vi "prop_axes_prop_to_page.vi"(10 "Axes Properties":T2) -> (2 "Axes Property Page":T1(array[cluster]))   [LabVIEW 2020, in "3DPC_SurfacePlot.xctl"]
uses:
  <vilib>/Native 3D Graph/xcontrol/3DPC_SurfacePlot.xctl
  <vilib>/Native 3D Graph/typedefs/prop_axes_all.ctl
  <vilib>/Native 3D Graph/typedefs/prop_axes_grid.ctl
  <vilib>/Native 3D Graph/typedefs/prop_axes_ticks.ctl
  <vilib>/Native 3D Graph/typedefs/range_cluster.ctl
  <vilib>/Native 3D Graph/typedefs/min_max.ctl
  <vilib>/Native 3D Graph/typedefs/prop_axes_captions.ctl
  <vilib>/Native 3D Graph/typedefs/prop_axes_labels.ctl
  <vilib>/Native 3D Graph/typedefs/prop_axes_autorange.ctl
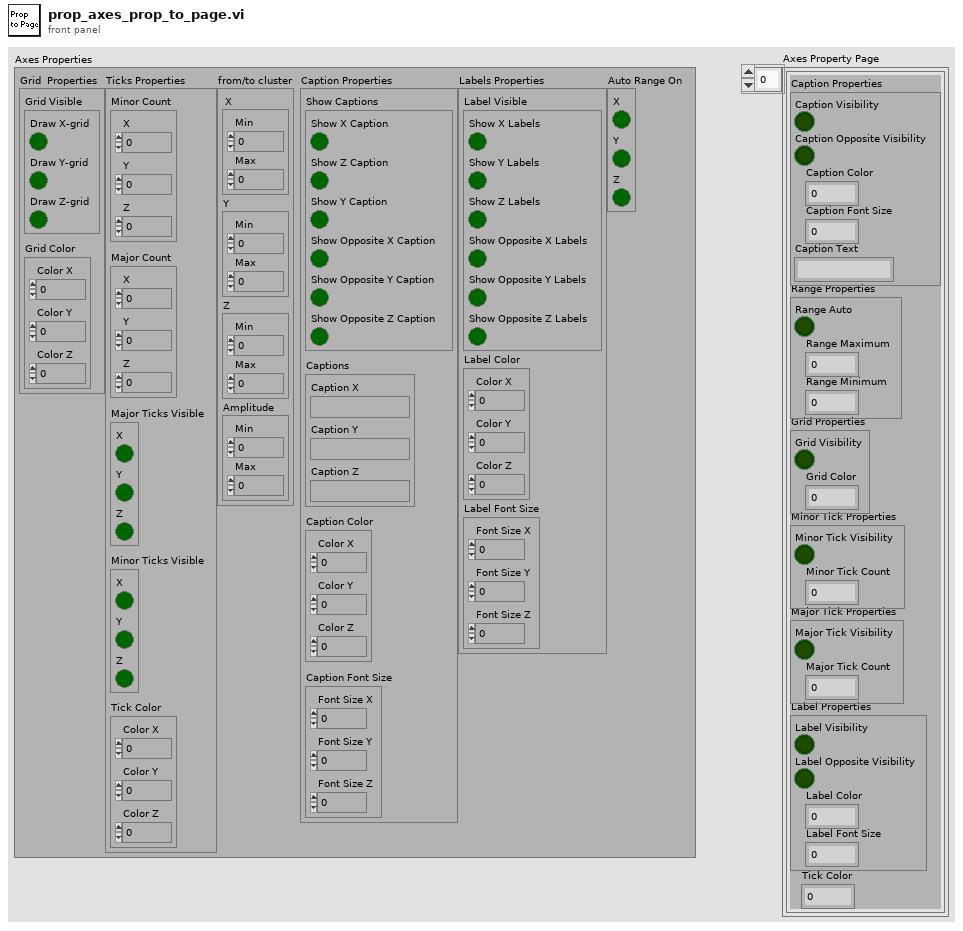
[diagram p1: front panel]
types:
  T1 = cluster{"Caption Properties":cluster{"Caption Visibility":bool, "Caption Opposite Visibility":bool, "Caption Color":u32, "Caption Font Size":i32, "Caption Text":string}, "Range Properties":cluster{"Range Auto":bool, "Range Maximum":dbl, "Range Minimum":dbl}, "Grid Properties":cluster{"Grid Visibility":bool, "Grid Color":u32}, "Minor Tick Properties":cluster{"Minor Tick Visibility":bool, "Minor Tick Count":i32}, "Major Tick Properties":cluster{"Major Tick Visibility":bool, "Major Tick Count":i32}, "Label Properties":cluster{"Label Visibility":bool, "Label Opposite Visibility":bool, "Label Color":u32, "Label Font Size":i32}, "Tick Color":u32}[]
  T2 = typedef "3DPC_SurfacePlot.xctl/prop_axes_all.ctl" = cluster{"Grid  Properties":T3, "Ticks Properties":T4, "from/to cluster":T5, "Caption Properties":T7, "Labels Properties":T8, "Auto Range On":T9}
  T3 = typedef "3DPC_SurfacePlot.xctl/prop_axes_grid.ctl" = cluster{"Grid Visible":cluster{"Draw X-grid":bool, "Draw Y-grid":bool, "Draw Z-grid":bool}, "Grid Color":cluster{"Color X":u32, "Color Y":u32, "Color Z":u32}}
  T4 = typedef "3DPC_SurfacePlot.xctl/prop_axes_ticks.ctl" = cluster{"Minor Count":cluster{"X":i32, "Y":i32, "Z":i32}, "Major Count":cluster{"X":i32, "Y":i32, "Z":i32}, "Major Ticks Visible":cluster{"X":bool, "Y":bool, "Z":bool}, "Minor Ticks Visible":cluster{"X":bool, "Y":bool, "Z":bool}, "Tick Color":cluster{"Color X":u32, "Color Y":u32, "Color Z":u32}}
  T5 = typedef "3DPC_SurfacePlot.xctl/range_cluster.ctl" = cluster{"X":T6, "Y":T6, "Z":T6, "Amplitude":T6}
  T6 = typedef "3DPC_SurfacePlot.xctl/min_max.ctl" = cluster{"Min":sgl, "Max":sgl}
  T7 = typedef "3DPC_SurfacePlot.xctl/prop_axes_captions.ctl" = cluster{"Show Captions":cluster{"Show X Caption":bool, "Show Z Caption":bool, "Show Y Caption":bool, "Show Opposite X Caption":bool, "Show Opposite Y Caption":bool, "Show Opposite Z Caption":bool}, "Captions":cluster{"Caption X":string, "Caption Y":string, "Caption Z":string}, "Caption Color":cluster{"Color X":u32, "Color Y":u32, "Color Z":u32}, "Caption Font Size":cluster{"Font Size X":i16, "Font Size Y":i16, "Font Size Z":i16}}
  T8 = typedef "3DPC_SurfacePlot.xctl/prop_axes_labels.ctl" = cluster{"Label Visible":cluster{"Show X Labels":bool, "Show Y Labels":bool, "Show Z Labels":bool, "Show Opposite X Labels":bool, "Show Opposite Y Labels":bool, "Show Opposite Z Labels":bool}, "Label Color":cluster{"Color X":u32, "Color Y":u32, "Color Z":u32}, "Label Font Size":cluster{"Font Size X":i16, "Font Size Y":i16, "Font Size Z":i16}}
  T9 = typedef "3DPC_SurfacePlot.xctl/prop_axes_autorange.ctl" = cluster{"X":bool, "Y":bool, "Z":bool}
  T10 = cluster{"Caption Properties":cluster{"Caption Visibility":bool, "Caption Opposite Visibility":bool, "Caption Color":u32, "Caption Font Size":i32, "Caption Text":string}, "Range Properties":cluster{"Range Auto":bool, "Range Maximum":dbl, "Range Minimum":dbl}, "Grid Properties":cluster{"Grid Visibility":bool, "Grid Color":u32}, "Minor Tick Properties":cluster{"Minor Tick Visibility":bool, "Minor Tick Count":i32}, "Major Tick Properties":cluster{"Major Tick Visibility":bool, "Major Tick Count":i32}, "Label Properties":cluster{"Label Visibility":bool, "Label Opposite Visibility":bool, "Label Color":u32, "Label Font Size":i32}, "Tick Color":u32}
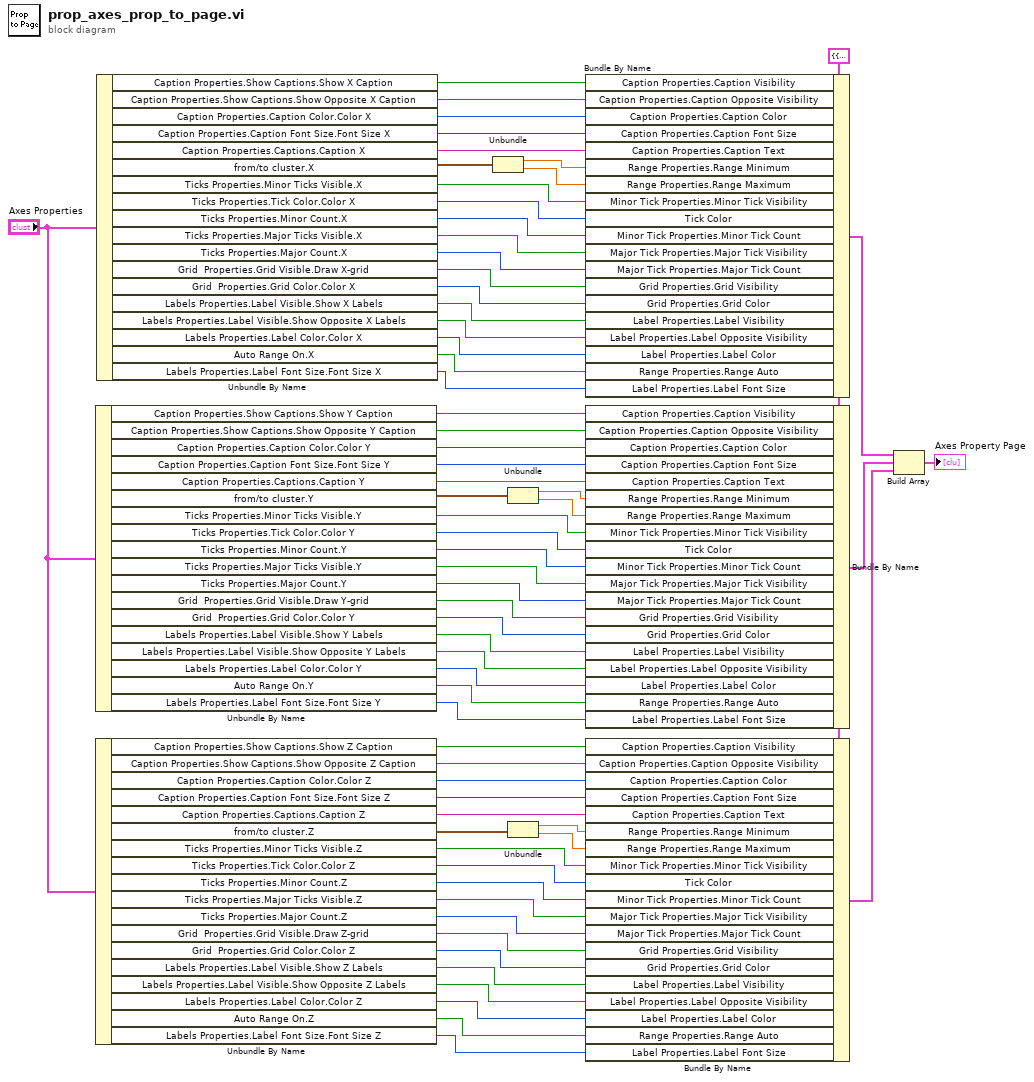
[diagram p0: block diagram]
diagram:
  w5 = T10 {"Caption Properties"={"Caption Visibility"=FALSE, "Caption Opposite Visibility"=FALSE, "Caption Color"=0, "Caption Font Size"=0, "Caption Text"=""}, "Range Properties"={"Range Auto"=FALSE, "Range Maximum"=0.0, "Range Minimum"=0.0}, "Grid Properties"={"Grid Visibility"=FALSE, "Grid Color"=0}, "Minor Tick Properties"={"Minor Tick Visibility"=FALSE, "Minor Tick Count"=0}, "Major Tick Properties"={"Major Tick Visibility"=FALSE, "Major Tick Count"=0}, "Label Properties"={"Label Visibility"=FALSE, "Label Opposite Visibility"=FALSE, "Label Color"=0, "Label Font Size"=0}, "Tick Color"=0} ("output cluster")
  n1 = Unbundle By Name("Axes Properties") -> ("Caption Properties.Show Captions.Show Y Caption"=w51:bool, "Caption Properties.Show Captions.Show Opposite Y Caption"=w16:bool, "Caption Properties.Caption Color.Color Y"=w50:u32, "Caption Properties.Caption Font Size.Font Size Y"=w49:i16, "Caption Properties.Captions.Caption Y"=w48:string, "from/to cluster.Y"=w47:T6, "Ticks Properties.Minor Ticks Visible.Y"=w44:bool, "Ticks Properties.Tick Color.Color Y"=w43:u32, "Ticks Properties.Minor Count.Y"=w42:i32, "Ticks Properties.Major Ticks Visible.Y"=w41:bool, "Ticks Properties.Major Count.Y"=w40:i32, "Grid  Properties.Grid Visible.Draw Y-grid"=w39:bool, "Grid  Properties.Grid Color.Color Y"=w9:u32, "Labels Properties.Label Visible.Show Y Labels"=w38:bool, "Labels Properties.Label Visible.Show Opposite Y Labels"=w2:bool, "Labels Properties.Label Color.Color Y"=w12:u32, "Auto Range On.Y"=w13:bool, "Labels Properties.Label Font Size.Font Size Y"=w6:i16)
  n2 = Unbundle By Name("Axes Properties") -> ("Caption Properties.Show Captions.Show Z Caption"=w37:bool, "Caption Properties.Show Captions.Show Opposite Z Caption"=w15:bool, "Caption Properties.Caption Color.Color Z"=w36:u32, "Caption Properties.Caption Font Size.Font Size Z"=w35:i16, "Caption Properties.Captions.Caption Z"=w34:string, "from/to cluster.Z"=w33:T6, "Ticks Properties.Minor Ticks Visible.Z"=w30:bool, "Ticks Properties.Tick Color.Color Z"=w29:u32, "Ticks Properties.Minor Count.Z"=w28:i32, "Ticks Properties.Major Ticks Visible.Z"=w27:bool, "Ticks Properties.Major Count.Z"=w26:i32, "Grid  Properties.Grid Visible.Draw Z-grid"=w25:bool, "Grid  Properties.Grid Color.Color Z"=w24:u32, "Labels Properties.Label Visible.Show Z Labels"=w23:bool, "Labels Properties.Label Visible.Show Opposite Z Labels"=w1:bool, "Labels Properties.Label Color.Color Z"=w10:u32, "Auto Range On.Z"=w11:bool, "Labels Properties.Label Font Size.Font Size Z"=w7:i16)
  n3 = Unbundle By Name("Axes Properties") -> ("Caption Properties.Show Captions.Show X Caption"=w66:bool, "Caption Properties.Show Captions.Show Opposite X Caption"=w17:bool, "Caption Properties.Caption Color.Color X"=w65:u32, "Caption Properties.Caption Font Size.Font Size X"=w64:i16, "Caption Properties.Captions.Caption X"=w63:string, "from/to cluster.X"=w62:T6, "Ticks Properties.Minor Ticks Visible.X"=w59:bool, "Ticks Properties.Tick Color.Color X"=w58:u32, "Ticks Properties.Minor Count.X"=w57:i32, "Ticks Properties.Major Ticks Visible.X"=w56:bool, "Ticks Properties.Major Count.X"=w55:i32, "Grid  Properties.Grid Visible.Draw X-grid"=w4:bool, "Grid  Properties.Grid Color.Color X"=w54:u32, "Labels Properties.Label Visible.Show X Labels"=w53:bool, "Labels Properties.Label Visible.Show Opposite X Labels"=w18:bool, "Labels Properties.Label Color.Color X"=w52:u32, "Auto Range On.X"=w14:bool, "Labels Properties.Label Font Size.Font Size X"=w8:i16)
  n4 = Unbundle(w62) -> ("Min"=w61:sgl, "Max"=w60:sgl)
  n5 = Unbundle(w47) -> ("Min"=w46:sgl, "Max"=w45:sgl)
  n6 = Unbundle(w33) -> ("Min"=w32:sgl, "Max"=w31:sgl)
  n7 = Bundle By Name(cluster=w5, "Caption Properties.Caption Visibility"=w66, "Caption Properties.Caption Opposite Visibility"=w17, "Caption Properties.Caption Color"=w65, "Caption Properties.Caption Font Size"=w64, "Caption Properties.Caption Text"=w63, "Range Properties.Range Minimum"=w61, "Range Properties.Range Maximum"=w60, "Minor Tick Properties.Minor Tick Visibility"=w59, "Tick Color"=w58, "Minor Tick Properties.Minor Tick Count"=w57, "Major Tick Properties.Major Tick Visibility"=w56, "Major Tick Properties.Major Tick Count"=w55, "Grid Properties.Grid Visibility"=w4, "Grid Properties.Grid Color"=w54, "Label Properties.Label Visibility"=w53, "Label Properties.Label Opposite Visibility"=w18, "Label Properties.Label Color"=w52, "Range Properties.Range Auto"=w14, "Label Properties.Label Font Size"=w8) -> (w22:T10)
  n8 = Bundle By Name(cluster=w5, "Caption Properties.Caption Visibility"=w51, "Caption Properties.Caption Opposite Visibility"=w16, "Caption Properties.Caption Color"=w50, "Caption Properties.Caption Font Size"=w49, "Caption Properties.Caption Text"=w48, "Range Properties.Range Minimum"=w46, "Range Properties.Range Maximum"=w45, "Minor Tick Properties.Minor Tick Visibility"=w44, "Tick Color"=w43, "Minor Tick Properties.Minor Tick Count"=w42, "Major Tick Properties.Major Tick Visibility"=w41, "Major Tick Properties.Major Tick Count"=w40, "Grid Properties.Grid Visibility"=w39, "Grid Properties.Grid Color"=w9, "Label Properties.Label Visibility"=w38, "Label Properties.Label Opposite Visibility"=w2, "Label Properties.Label Color"=w12, "Range Properties.Range Auto"=w13, "Label Properties.Label Font Size"=w6) -> (w21:T10)
  n9 = Bundle By Name(cluster=w5, "Caption Properties.Caption Visibility"=w37, "Caption Properties.Caption Opposite Visibility"=w15, "Caption Properties.Caption Color"=w36, "Caption Properties.Caption Font Size"=w35, "Caption Properties.Caption Text"=w34, "Range Properties.Range Minimum"=w32, "Range Properties.Range Maximum"=w31, "Minor Tick Properties.Minor Tick Visibility"=w30, "Tick Color"=w29, "Minor Tick Properties.Minor Tick Count"=w28, "Major Tick Properties.Major Tick Visibility"=w27, "Major Tick Properties.Major Tick Count"=w26, "Grid Properties.Grid Visibility"=w25, "Grid Properties.Grid Color"=w24, "Label Properties.Label Visibility"=w23, "Label Properties.Label Opposite Visibility"=w1, "Label Properties.Label Color"=w10, "Range Properties.Range Auto"=w11, "Label Properties.Label Font Size"=w7) -> (w20:T10)
  n10 = Build Array(w22, w21, w20) -> (→"Axes Property Page":T1)
